vi "ALapp_I_term.vi"(2 "I Term Gain":dbl, 3 "error":dbl) -> (0 "I Term Output":dbl)   [LabVIEW 2011]
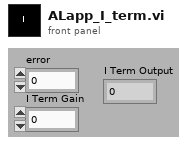
[diagram p1: front panel]
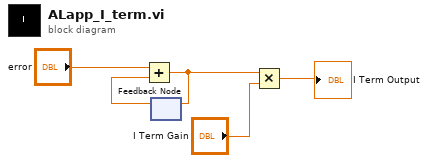
[diagram p0: block diagram]
diagram:
  n1 = feedback #1() -> (w4:dbl)  [unwired: 1 out]
  n2 = Add(x="error", y=w4) -> (x+y=w3:dbl)
  n3 = feedback-in #1(w3) -> ()
  n4 = Multiply(x=w3, y="I Term Gain") -> (x*y=→"I Term Output":dbl)
